vi "subLocateStatus.vi"(1 "Value":dbl format="%#_13g", 2 "parameter":T1) -> (0 "Status":i32)   [LabVIEW 2014]
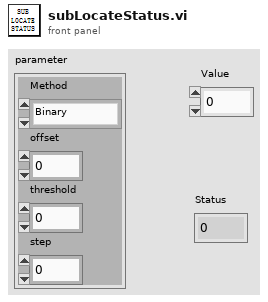
[diagram p1: front panel]
types:
  T1 = cluster{"Method":enum16{"Binary", "Uniform"}, "offset":i32, "threshold":dbl, "step":dbl}
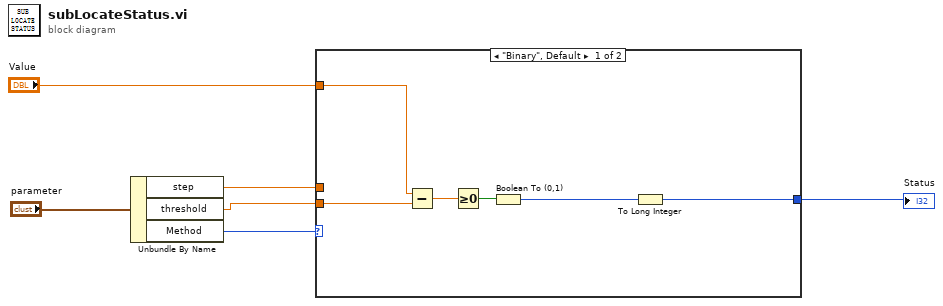
[diagram p0: block diagram]
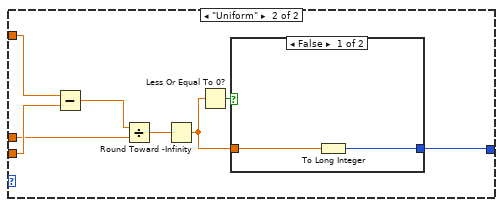
[diagram p2: hidden frame]
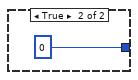
[diagram p3: hidden frame]
diagram:
  n1 = Unbundle By Name("parameter") -> ("step"=w2:dbl, "threshold"=w3:dbl, "Method"=w5:enum16{"Binary", "Uniform"})
  n2 = case shown="\"Binary\", Default" w5 {
    tunnel: "Value" -> [w12 w20]
    tunnel: w3 -> [w11 w19]
    tunnel: [w7 w14] -> w1
    tunnel: w2 -> [_ w18]
    frame "Binary", Default {
      n3 = Subtract(x=w12, y=w11) -> (x-y=w10:dbl)
      n4 = Greater Or Equal To 0?(x=w10) -> (x >= 0?=w9:bool)
      n5 = Boolean To (0,1)(Boolean=w9) -> (0, 1=w8:i16)
      n6 = To Long Integer(number=w8) -> (32bit integer=w7:i32)
    }
    frame "Uniform" {
      n7 = Subtract(x=w20, y=w19) -> (x-y=w17:dbl)
      n8 = Divide(x=w17, y=w18) -> (x/y=w16:dbl)
      n9 = Round Toward -Infinity(1:w16) -> (0:w13:dbl)
      n10 = Less Or Equal To 0?(x=w13) -> (x <= 0?=w15:bool)
      n11 = case shown="False" w15 {
        tunnel: [w21 0] -> w14
        tunnel: w13 -> [w22 _]
        frame False {
          n12 = To Long Integer(number=w22) -> (32bit integer=w21:i32)
        }
        frame True {
        }
      }
    }
  }
  "Status" <- w1
